vi "Get Address.vi"(8 "error in (no error)":errorcluster, 11 "RRG in":refnum<class "Eltochpribor RRG.lvclass">) -> (0 "error out":errorcluster, 2 "address":u8, 3 "RRG out":refnum<class "Eltochpribor RRG.lvclass">)   [LabVIEW 2015, in "Eltochpribor RRG.lvclass"]
doc: "Gets communication address."
uses:
  Eltochpribor RRG.lvclass
  Modbus Client/PL Modbus Client.lvclass
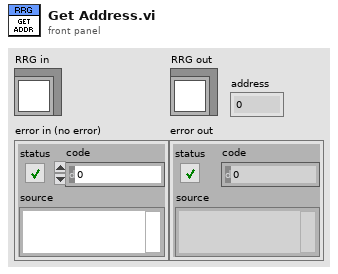
[diagram p1: front panel]
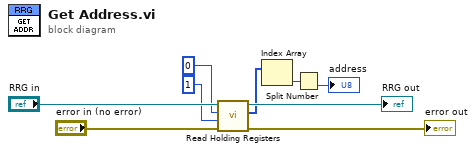
[diagram p0: block diagram]
diagram:
  n1 = call "Read Holding Registers.vi"("error in (no error)"="error in (no error)", "number of holding registers"=u16 1, "address"=u16 0, "MODBUS in"="RRG in") -> ("error out"=→"error out":errorcluster, "values"=w3:u16[], "MODBUS out"=→"RRG out":refnum<class "Eltochpribor RRG.lvclass">)  [unwired: 5 in]
  n2 = Index Array(array=w3) -> (element=w2:u16)  [unwired: 1 in]
  n3 = Split Number(x=w2) -> (lo(x)=→"address":u8)  [unwired: 1 out]
